vi "ArrDevMeasAction.vi"(7 "DevId":i32, 8 "error in (no error)":errorcluster caption="entrée d'erreur (pas d'erreur)", 9 "CurvePointIndex":i32, 10 "AllPointIndex":i32, 11 "Device In":refnum<class "SymphonyCCD.lvclass"> caption="DNL_LabVIEW Object in") -> (0 "error out":errorcluster caption="sortie d'erreur", 1 "ArrDevDat":T1[](array[typedef]), 2 "ArrDevDatOut":dbl[][](array[numeric]), 3 "Device Out":refnum<class "SymphonyCCD.lvclass"> caption="DNL_LabVIEW Object out", 5 "MeasOut":dbl[](array[numeric]))   [LabVIEW 2019, in "SymphonyCCD.lvclass"]
uses:
  SymphonyCCD.lvclass
  C:/Programmes Labview/LabScanV1A/DevicesClass/BaseDevice/BaseDevice.lvclass
  Experiment Class/ArrDevData.ctl
  SymphonyCCD.lvclass/SymphonyCCD.ctl
  <userlib>/JY Symphony/NoiseCorr.ctl
  <userlib>/GenProg/ReadValByRefBool.vi
  <userlib>/GenProg/ReadValByRefDbl.vi
  <userlib>/GenProg/ReadValByRefU32.vi
  <userlib>/GenProg/ReadValByRefU16.vi
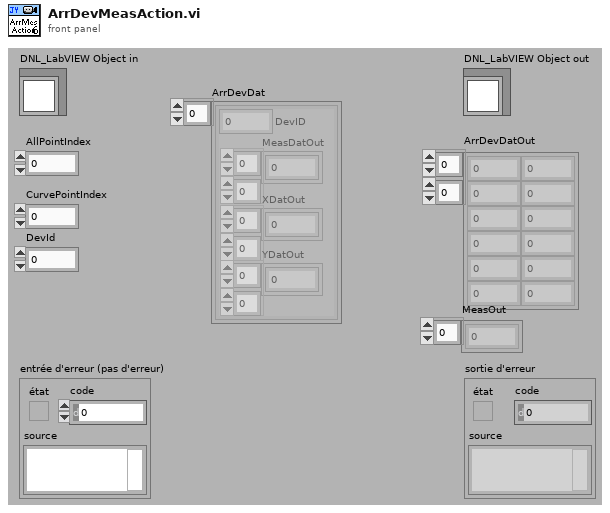
[diagram p1: front panel]
types:
  T1 = typedef "ArrDevData.ctl" = cluster{"MeasDatOut":dbl[][], "XDatOut":dbl[][], "YDatOut":dbl[][], "DevID":i32}
  T2 = typedef "NoiseCorr.ctl" = enum16{"Off", "One For All Acq", "One For Every Acq"}
  T3 = cluster{"Message":string, "Data":variant, "Code":i32}
  T4 = typedef "SymphonyCCD.lvclass/SymphonyCCD_Func.ctl" = enum16{"AcqImageSim (Counts)", "AcqImage (Counts)"}
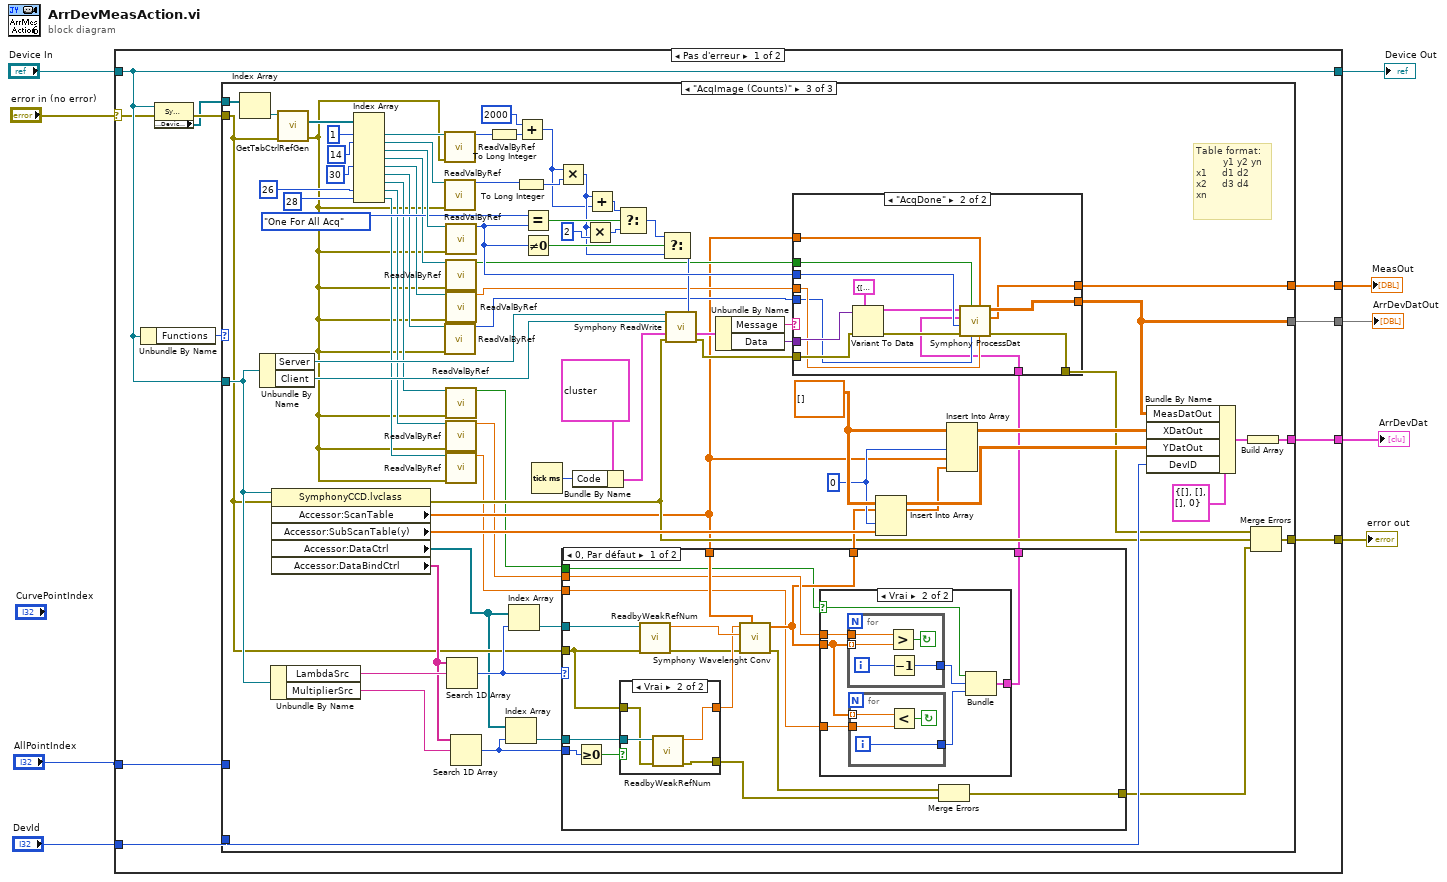
[diagram p0: block diagram]
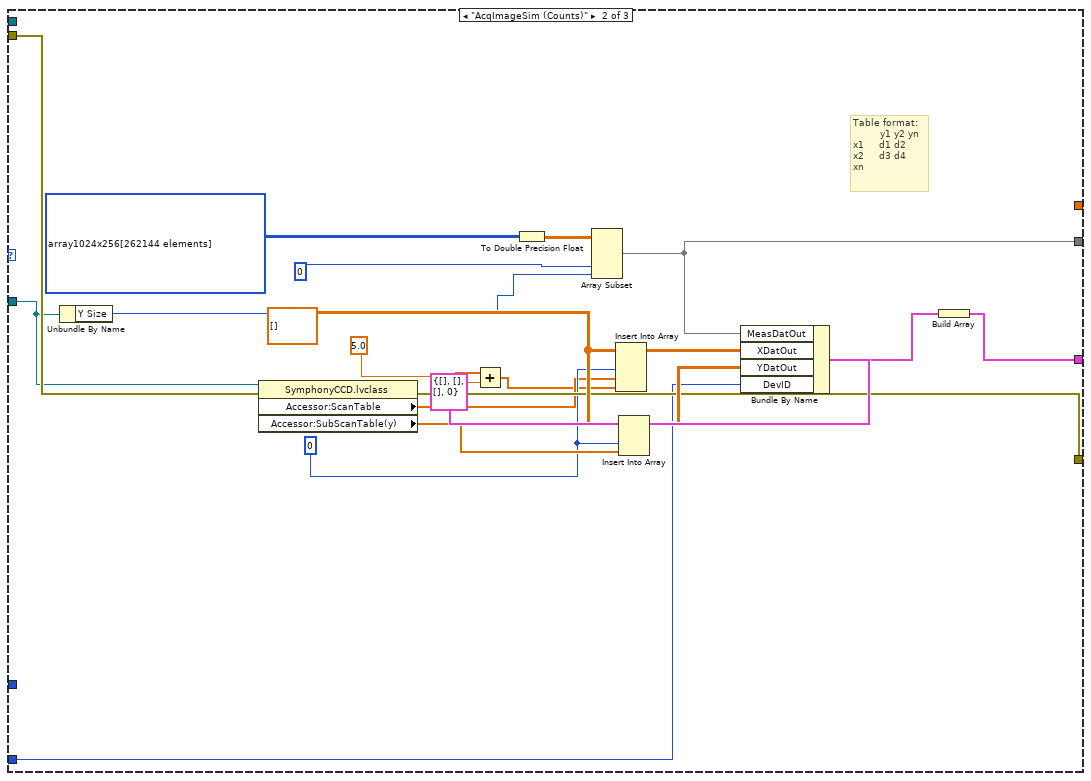
[diagram p3: hidden frame]
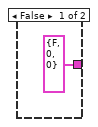
[diagram p4: hidden frame]
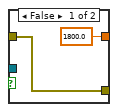
[diagram p5: hidden frame]
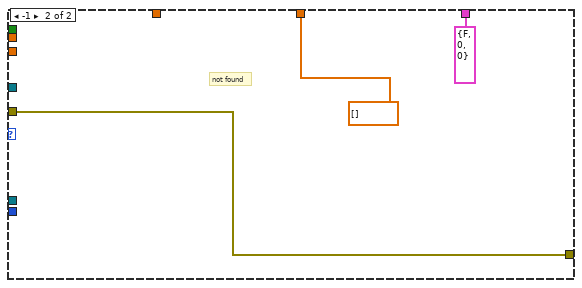
[diagram p6: hidden frame]
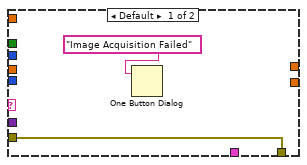
[diagram p7: hidden frame]
diagram:
  n1 = case shown="Pas d'erreur" "error in (no error)" {
    selector: "error in (no error)" -> [w13 w179]
    tunnel: [w16 w179] -> w9
    tunnel: [w14 w178] -> w7
    tunnel: "Device In" -> [w14 w178]
    tunnel: [w18 _] -> w8
    tunnel: "AllPointIndex" -> [w19 _]
    tunnel: [w17 _] -> w3
    tunnel: "DevId" -> [w15 _]
    tunnel: [w10 _] -> w1
    frame No Error {
      n2 = Unbundle By Name(w14) -> ("Functions"=w20:T4)
      n3 = property class="SymphonyCCD.lvclass"(reference=w14, error in=w13) -> (error out=w12:errorcluster, "Accessor:DeviceCtrl"=w11:refnum<vi>[])  [unwired: 1 out]
      n4 = case shown="\"AcqImage (Counts)\"" w20 {
        tunnel: w19 -> [_ _ _]
        tunnel: [_ w27 w100] -> w18
        tunnel: w14 -> [_ w30 w97]
        tunnel: [_ w34 w112] -> w17
        tunnel: w12 -> [w21 w33 w82]
        tunnel: [w21 w32 w99] -> w16
        tunnel: w15 -> [_ w25 w110]
        tunnel: w11 -> [_ _ w77]
        tunnel: [_ _ w55] -> w10
        frame Default {
        }
        frame "AcqImageSim (Counts)" {
          w31 = 0 ("indice désactivé (col)")
          w35 = dbl[][] [] ("tableau")
          # "Table format: \n         y1 y2 yn\nx1     d1 d2\nx2     d3 d4\nxn"
          n5 = Unbundle By Name(w30) -> ("Y Size"=w26:i32)
          n6 = property class="SymphonyCCD.lvclass"(reference=w30, error in=w33) -> (error out=w32:errorcluster, "Accessor:ScanTable"=w24:dbl[], "Accessor:SubScanTable(y)"=w36:dbl[])  [unwired: 1 out]
          n7 = Add(x=w24, y=5.0) -> (x+y=w22:dbl[])
          n8 = To Double Precision Float(number=i32[][] array1024x256[262144 elements]) -> (double precision float=w29:dbl[][])
          n9 = Array Subset(array=w29, index (col)=0 ("indice"), length (col)=w26) -> (w27:dbl[][])  [unwired: 2 in]
          n10 = Insert Into Array(array=w35, index (col)=w31, new element #1=w24, new element #2=w22) -> (w38:dbl[][])  [unwired: 1 in]
          n11 = Insert Into Array(array=w35, index (col)=w31, new element=w36) -> (w37:dbl[][])  [unwired: 1 in]
          n12 = Bundle By Name(cluster=T1 {"MeasDatOut"=[], "XDatOut"=[], "YDatOut"=[], "DevID"=0} ("cluster de sortie"), "MeasDatOut"=w27, "XDatOut"=w38, "YDatOut"=w37, "DevID"=w25) -> (w39:T1)
          n13 = Build Array(w39) -> (w34:T1[])
        }
        frame "AcqImage (Counts)" {
          w111 = 0 ("indice désactivé (col)")
          w113 = dbl[][] [] ("tableau")
          # "Table format: \n         y1 y2 yn\nx1     d1 d2\nx2     d3 d4\nxn"
          n14 = Index Array(array=w77) -> (element=w87:refnum<vi>)  [unwired: 1 in]
          n15 = Unbundle By Name(w97) -> ("Server"=w109:refnum<k13>, "Client"=w108:refnum<k13>)
          n16 = Unbundle By Name(w97) -> ("LambdaSrc"=w96:string, "MultiplierSrc"=w92:string)
          n17 = property class="SymphonyCCD.lvclass"(reference=w97, error in=w82) -> (error out=w59:errorcluster, "Accessor:ScanTable"=w54:dbl[], "Accessor:SubScanTable(y)"=w114:dbl[], "Accessor:DataCtrl"=w50:refnum<vi>[], "Accessor:DataBindCtrl"=w91:string[])  [unwired: 1 out]
          n18 = call <userlib>:"GetTabCtrlRefGen.vi"("ErrorIn(No Error)"=w82, "CommandRef"=w87) -> ("sortie d'erreur"=w44:errorcluster, "ControlsRefs"=w86:refnum<vi>[])  [unwired: 7 in, 1 out]
          n19 = Index Array(array=w86, index #1=1 ("index"), index #2=14 ("indice"), index #5=30 ("index"), index #8=26 ("index"), index #9=28 ("index")) -> (element #1=w84:refnum<vi>, element #2=w81:refnum<vi>, element #3=w78:refnum<vi>, element #4=w62:refnum<vi>, element #5=w60:refnum<vi>, element #6=w53:refnum<vi>, element #7=w45:refnum<vi>, element #8=w47:refnum<vi>, element #9=w52:refnum<vi>)  [unwired: 4 in]
          n20 = call-poly <userlib>:"ReadValByRef.vi"("Control Ref"=w84, "error in"=w44) -> ("Valeur"=w83:u32)  [unwired: 12 in, 1 out]
          n21 = call-poly <userlib>:"ReadValByRef.vi"("Control Ref"=w81, "error in"=w44) -> ("Valeur"=w79:u16)  [unwired: 12 in, 1 out]
          n22 = call-poly <userlib>:"ReadValByRef.vi"("Control Ref"=w53, "error in"=w44) -> ("Valeur"=w56:u32)  [unwired: 12 in, 1 out]
          n23 = call-poly <userlib>:"ReadValByRef.vi"("Control Ref"=w78, "error in"=w44) -> ("Valeur"=w73:u16)  [unwired: 12 in, 1 out]
          n24 = call-poly <userlib>:"ReadValByRef.vi"("Control Ref"=w62, "error in"=w44) -> ("Valeur"=w61:bool)  [unwired: 12 in, 1 out]
          n25 = call-poly <userlib>:"ReadValByRef.vi"("Control Ref"=w60, "error in"=w44) -> ("Valeur"=w57:dbl)  [unwired: 12 in, 1 out]
          n26 = call-poly <userlib>:"ReadValByRef.vi"("Control Ref"=w45, "error in"=w44) -> ("Valeur"=w43:bool)  [unwired: 12 in, 1 out]
          n27 = call-poly <userlib>:"ReadValByRef.vi"("Control Ref"=w47, "error in"=w44) -> ("Valeur"=w51:dbl)  [unwired: 12 in, 1 out]
          n28 = call-poly <userlib>:"ReadValByRef.vi"("Control Ref"=w52, "error in"=w44) -> ("Valeur"=w49:dbl)  [unwired: 12 in, 1 out]
          n29 = Search 1D Array(1D array=w91, element=w96) -> (index of element=w93:i32)  [unwired: 1 in]
          n30 = Search 1D Array(1D array=w91, element=w92) -> (index of element=w90:i32)  [unwired: 1 in]
          n31 = To Long Integer(number=w83) -> (32bit integer=w65:i32)
          n32 = Index Array(array=w50, index=w90) -> (element=w89:refnum<vi>)
          n33 = Index Array(array=w50, index=w93) -> (element=w95:refnum<vi>)
          n34 = To Long Integer(number=w79) -> (32bit integer=w66:i32)
          n35 = Add(x=2000, y=w65) -> (x+y=w63:i32)
          n36 = Equal?(x=NoiseCorr."One For All Acq" ("Valeur"), y=w73) -> (x = y?=w72:bool)
          n37 = Not Equal To 0?(x=w73) -> (x != 0?=w76:bool)
          n38 = Tick Count (ms)() -> (millisecond timer value=w105:u32)
          n39 = Multiply(x=w63, y=w66) -> (x*y=w67:i32)
          n40 = case shown="0, Par défaut" w93 {
            tunnel: w54 -> [w128 _]
            tunnel: w82 -> [w133 w160]
            tunnel: w95 -> [w135 _]
            tunnel: [w122 dbl[] []] -> w94
            tunnel: w90 -> [w129 _]
            tunnel: w89 -> [w134 _]
            tunnel: [w131 w160] -> w88
            tunnel: w51 -> [w123 _]
            tunnel: w49 -> [w121 _]
            tunnel: w43 -> [w120 _]
            tunnel: [w119 cluster{bool, i32, i32} {FALSE, 0, 0}] -> w42
            frame 0, Default {
              n41 = Greater Or Equal To 0?(x=w129) -> (x >= 0?=w130:bool)
              n42 = case shown="Vrai" w130 {
                tunnel: w134 -> [_ w158]
                tunnel: w133 -> [w153 w157]
                tunnel: [w153 w156] -> w132
                tunnel: [1800.0 ("Valeur") w155] -> w126
                frame False {
                }
                frame True {
                  n43 = call <userlib>:"ReadbyWeakRefNum.vi"("error in"=w157, "Control Ref"=w158) -> ("error out"=w156:errorcluster, "Valeur"=w155:dbl)  [unwired: 8 in]
                }
              }
              n44 = call <userlib>:"ReadbyWeakRefNum.vi"("error in"=w133, "Control Ref"=w135) -> ("error out"=w125:errorcluster, "Valeur"=w127:dbl)  [unwired: 8 in]
              n45 = call <userlib>:"Symphony Wavelenght Conv.vi"("PixelArr"=w128, "error in (no error)"=w125, "Lambda"=w127, "Grooves(l/mm)"=w126) -> ("error out"=w124:errorcluster, "Tableau"=w122:dbl[])  [unwired: 6 in]
              n46 = case shown="Vrai" w120 {
                selector: w120 -> [_ w139]
                tunnel: w123 -> [_ w143]
                tunnel: w122 -> [_ w137]
                tunnel: w121 -> [_ w142]
                tunnel: [cluster{bool, i32, i32} {FALSE, 0, 0} w138] -> w119
                frame False {
                }
                frame True {
                  n47 = for {
                    tunnel: w137 -> [w151] mode=indexing
                    tunnel: w143 -> [w152]
                    tunnel: [w148] -> w141
                    i -> [w149]
                    stop <- w150 continue-if-true
                    n48 = Greater?(x=w152, y=w151) -> (0:w150:bool)
                    n49 = Decrement(x=w149) -> (x-1=w148:i32)
                  }
                  n50 = for {
                    tunnel: w137 -> [w145] mode=indexing
                    tunnel: w142 -> [w146]
                    tunnel: [w144] -> w140
                    i -> [w144]
                    stop <- w147 continue-if-true
                    n51 = Less?(x=w145, y=w146) -> (x < y?=w147:bool)
                  }
                  n52 = Bundle(w139, w141, w140) -> (w138:cluster{bool, i32, i32})  [unwired: 1 in]
                }
              }
              n53 = Merge Errors(w124, w132) -> (w131:errorcluster)
            }
            frame -1 {
              # "not found"
            }
          }
          n54 = Bundle By Name(cluster=T3 {"Message"="AcqImage", "Data"=variant, "Code"=0} ("Message In"), "Code"=w105) -> (w106:T3)
          n55 = Multiply(x=w67, y=2 ("Read timeout ms(10000)")) -> (x*y=w68:i32)
          n56 = Add(x=w67, y=w63) -> (x+y=w71:i32)
          n57 = Select(t=w71, s=w72, f=w68) -> (s? t:f=w75:i32)
          n58 = Select(t=w75, s=w76, f=w67) -> (s? t:f=w70:i32)
          n59 = call <userlib>:"Symphony ReadWrite.vi"("ServerIn"=w109, "Read timeout ms(10000)"=w70, "ClientIn"=w108, "Message In"=w106, "ErrorIn (no error)"=w59) -> ("Data Out"=w104:T3, "error out"=w101:errorcluster)  [unwired: 7 in, 2 out]
          n60 = Unbundle By Name(w104) -> ("Message"=w103:string, "Data"=w102:variant)
          n61 = case shown="\"AcqDone\"" w103 {
            tunnel: w102 -> [_ w175]
            tunnel: w101 -> [w162 w177]
            tunnel: [_ w173] -> w100
            tunnel: [w162 w172] -> w98
            tunnel: w73 -> [_ w171]
            tunnel: w61 -> [_ w170]
            tunnel: w57 -> [_ w169]
            tunnel: w56 -> [_ w168]
            tunnel: [_ w167] -> w55
            tunnel: w54 -> [_ w166]
            tunnel: w42 -> [_ w164]
            frame Default {
              n62 = One Button Dialog(message="Image Acquisition Failed") -> ()  [unwired: 1 in, 1 out]
            }
            frame "AcqDone" {
              n63 = Variant To Data(error in=w177, type=cluster{i32[][][], dbl, bool} {[], 0.0, TRUE}, Variant=w175) -> (data=w165:cluster{i32[][][], dbl, bool}, error out=w174:errorcluster)
              n64 = call <userlib>:"Symphony ProcessDat.vi"("Window Width (ds)"=w169, "PixelArr"=w166, "Avg Samples"=w168, "Noise Window"=w170, "error in (no error)"=w174, "Noise Substract"=w171, "MaxFind"=w164, "DataIn"=w165) -> ("error out"=w172:errorcluster, "Max_and_Pix"=w167:dbl[], "TableauOut"=w173:dbl[][])  [unwired: 1 in]
            }
          }
          n65 = Insert Into Array(array=w113, index (col)=w111, new element=w114) -> (w115:dbl[][])  [unwired: 1 in]
          n66 = Insert Into Array(array=w113, index (col)=w111, new element #1=w54, new element #2=w94) -> (w116:dbl[][])  [unwired: 1 in]
          n67 = Bundle By Name(cluster=T1 {"MeasDatOut"=[], "XDatOut"=[], "YDatOut"=[], "DevID"=0} ("cluster de sortie"), "MeasDatOut"=w100, "XDatOut"=w116, "YDatOut"=w115, "DevID"=w110) -> (w117:T1)
          n68 = Build Array(w117) -> (w112:T1[])
          n69 = Merge Errors(w98, w59, w88) -> (w99:errorcluster)
        }
      }
    }
    frame Error {
    }
  }
  "error out" <- w9
  "Device Out" <- w7
  "ArrDevDatOut" <- w8
  "ArrDevDat" <- w3
  "MeasOut" <- w1
